vi "TTM.vi"() -> ()   [LabVIEW 2009]
doc: "This is the Target Temperature Monitoring module (TTM).\nIts job is to read all temperature measurement devices and report back the information."
uses:
  TTM Global.vi
panel:
  in  "Read LakeShore":bool
  in  "Read ITC4":bool
  in  "Read He4 Manometer":bool
  in  "Read He3 Manometer":bool
  in  "He4 Range":enum32{"X 1", "X 0.1", "X 0.01", "X 0.001"}(ring)=enum."X 0.01"
  in  "He3 Range":i32(ring)=2 items=["range X0.01", "range X0.1", "range X1"]
  out "TTM Message Type":T1(ring)=enum."He3Range="
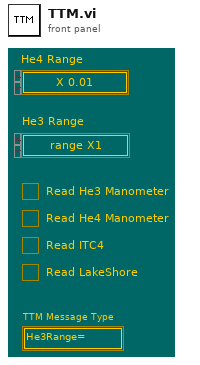
[diagram p1: front panel]
types:
  T1 = enum16{"No Message", "Bad Message", "He3Range=", "He4Range=", "GenEvent=", "Ping=", "Stop"}
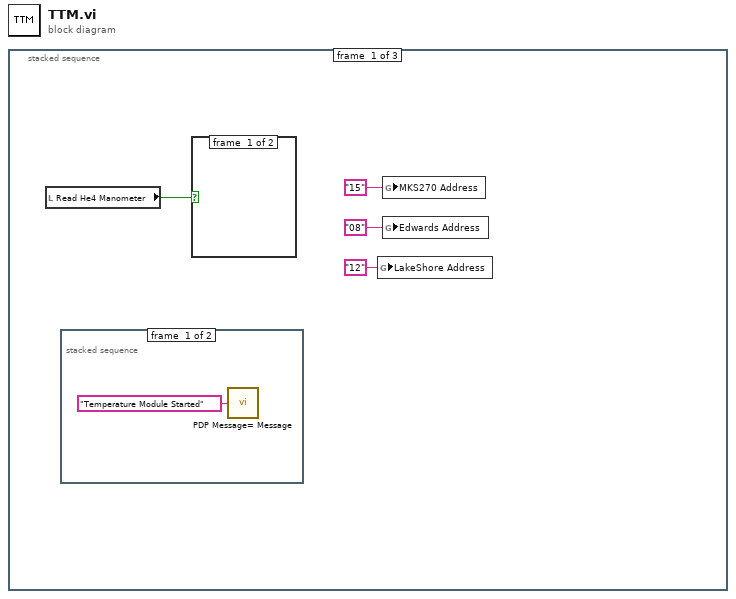
[diagram p0: block diagram]
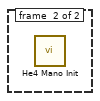
[diagram p2: hidden frame]
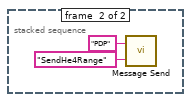
[diagram p3: hidden frame]
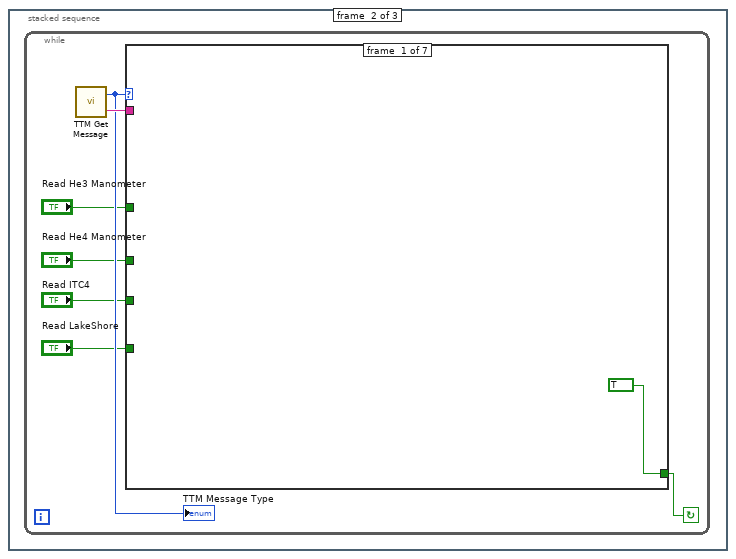
[diagram p4: hidden frame]
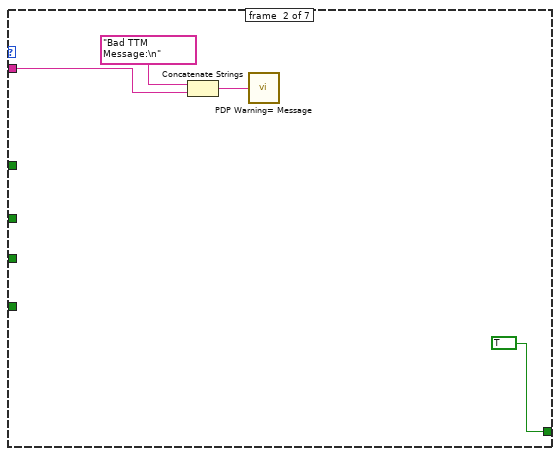
[diagram p5: hidden frame]
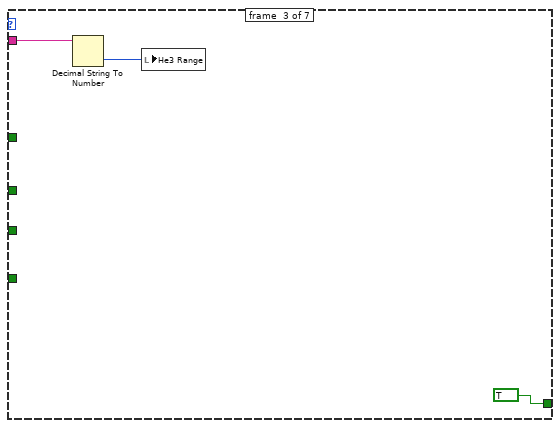
[diagram p6: hidden frame]
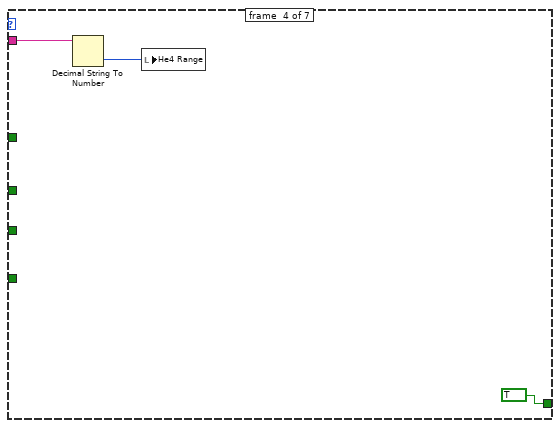
[diagram p7: hidden frame]
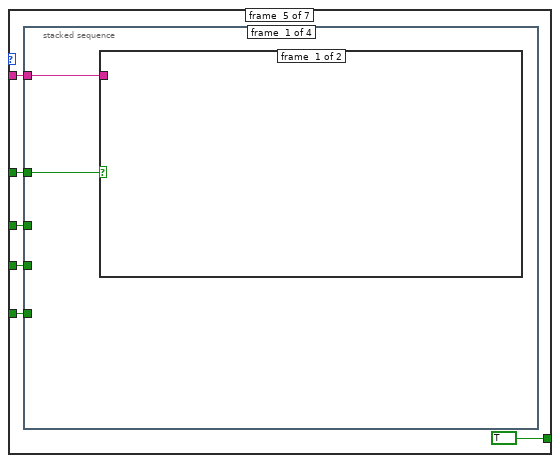
[diagram p8: hidden frame]
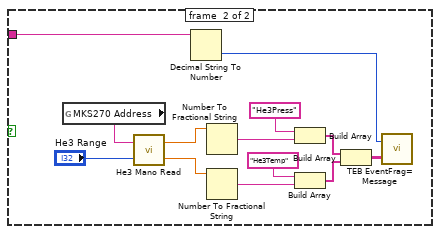
[diagram p9: hidden frame]
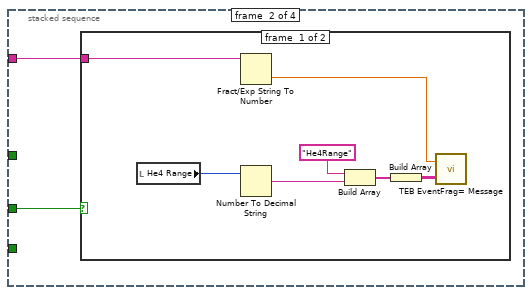
[diagram p10: hidden frame]
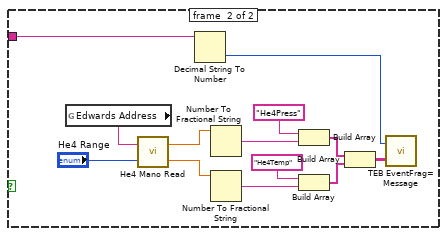
[diagram p11: hidden frame]
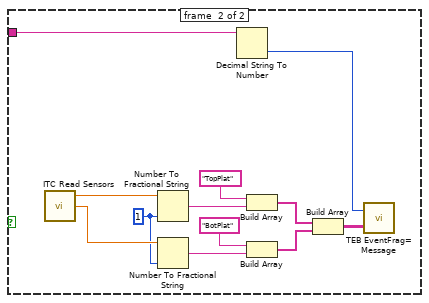
[diagram p13: hidden frame]
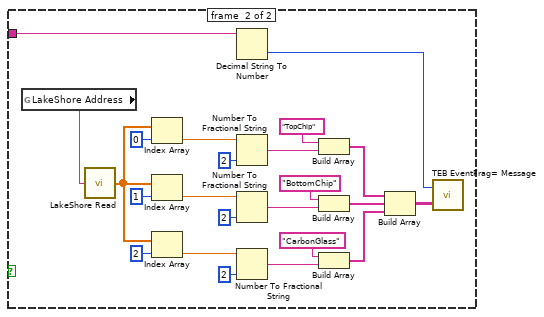
[diagram p15: hidden frame]
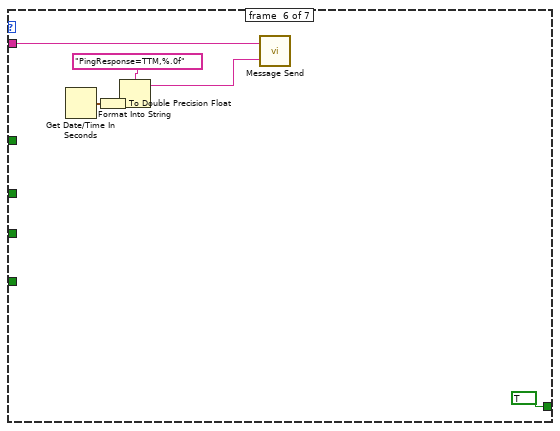
[diagram p16: hidden frame]
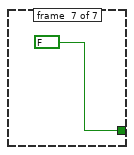
[diagram p17: hidden frame]
diagram:
  n1 = stacked-sequence {
    frame #0 {
      n2 = local read "Read He4 Manometer"() -> (w1:bool)
      n3 = stacked-sequence {
        frame #0 {
          n4 = call "PDP Message= Message.vi"("Message"="Temperature Module Started") -> ()
        }
        frame #1 {
          n5 = call "Message Send.vi"("Message"="SendHe4Range", "Destination"="PDP") -> ()
        }
      }
      n6 = case shown="True" w1 {
        frame #0 {
        }
        frame #1 {
          n7 = call "He4 Mano Init.vi"() -> ()  [unwired: 1 in]
        }
      }
      n8 = global write "TTM Global.vi" "LakeShore Address"("12" ("Edwards Address")) -> ()
      n9 = global write "TTM Global.vi" "MKS270 Address"("15" ("MKS270 Address")) -> ()
      n10 = global write "TTM Global.vi" "Edwards Address"("08" ("Edwards Address")) -> ()
    }
    frame #1 {
      n11 = while {
        stop <- w13 continue-if-true
        n12 = call "TTM Get Message.vi"() -> ("Text"=w14:string, "TTM Message Type"=w12:T1)
        "TTM Message Type" <- w12
        n13 = case shown="\"GenEvent=\"" w12 {
          tunnel: w14 -> [_ w19 w21 w24 w31 w109 _]
          tunnel: [TRUE TRUE TRUE TRUE TRUE TRUE FALSE] -> w13
          tunnel: "Read He3 Manometer" -> [_ _ _ _ w29 _ _]
          tunnel: "Read He4 Manometer" -> [_ _ _ _ w28 _ _]
          tunnel: "Read ITC4" -> [_ _ _ _ w27 _ _]
          tunnel: "Read LakeShore" -> [_ _ _ _ w26 _ _]
          frame #0 {
          }
          frame #1 {
            n14 = Concatenate Strings("Bad TTM Message:\n", w19) -> (w17:string)
            n15 = call "PDP Warning= Message.vi"("Message"=w17) -> ()
          }
          frame #2 {
            n16 = Decimal String To Number(string=w21) -> (number=w20:i32)  [unwired: 2 in, 1 out]
            n17 = local write "He3 Range"(w20) -> ()
          }
          frame #3 {
            n18 = Decimal String To Number(string=w24) -> (number=w23:i32)  [unwired: 2 in, 1 out]
            n19 = local write "He4 Range"(w23) -> ()
          }
          frame #4 {
            n20 = stacked-sequence {
              tunnel: w31 -> [w33 w48 w70 w84]
              tunnel: w29 -> [w32 _ _ _]
              tunnel: w28 -> [_ w47 _ _]
              tunnel: w27 -> [_ _ w69 _]
              tunnel: w26 -> [_ _ _ w83]
              frame #0 {
                n21 = case shown="True" w32 {
                  tunnel: w33 -> [_ w46]
                  frame #0 {
                  }
                  frame #1 {
                    n22 = global read "TTM Global.vi" "MKS270 Address"() -> (w35:string)
                    n23 = call "He3 Mano Read.vi"("Range"="He3 Range", "GPIB Address"=w35) -> ("3He Temp (K)"=w37:dbl, "3He Pressure (Torr)"=w36:dbl)
                    n24 = Decimal String To Number(string=w46) -> (number=w45:i32)  [unwired: 2 in, 1 out]
                    n25 = Number To Fractional String(number=w36) -> (F-format string=w38:string)  [unwired: 3 in]
                    n26 = Number To Fractional String(number=w37) -> (F-format string=w42:string)  [unwired: 3 in]
                    n27 = Build Array("He3Press", w38) -> (w39:string[])
                    n28 = Build Array("He3Temp", w42) -> (w43:string[])
                    n29 = Build Array(w39, w43) -> (w44:string[][])
                    n30 = call "TEB EventFrag= Message.vi"("Event Fragment(s)"=w44, "Event Number"=w45) -> ()
                  }
                }
              }
              frame #1 {
                n31 = case shown="True" w47 {
                  tunnel: w48 -> [w52 w68]
                  frame #0 {
                    n32 = local read "He4 Range"() -> (w50:enum32{"X 1", "X 0.1", "X 0.01", "X 0.001"})
                    n33 = Fract/Exp String To Number(string=w52) -> (number=w53:dbl)  [unwired: 3 in, 1 out]
                    n34 = Number To Decimal String(number=w50) -> (decimal integer string=w49:string)  [unwired: 1 in]
                    n35 = Build Array("He4Range", w49) -> (w55:string[])
                    n36 = Build Array(w55) -> (w51:string[][])
                    n37 = call "TEB EventFrag= Message.vi"("Event Fragment(s)"=w51, "Event Number"=w53) -> ()
                  }
                  frame #1 {
                    n38 = global read "TTM Global.vi" "Edwards Address"() -> (w57:string)
                    n39 = call "He4 Mano Read.vi"("Range"="He4 Range", "GPIB Address"=w57) -> ("Temperature (K)"=w59:dbl, "Vapor pressure (torr)"=w58:dbl)
                    n40 = Decimal String To Number(string=w68) -> (number=w67:i32)  [unwired: 2 in, 1 out]
                    n41 = Number To Fractional String(number=w58) -> (F-format string=w60:string)  [unwired: 3 in]
                    n42 = Number To Fractional String(number=w59) -> (F-format string=w64:string)  [unwired: 3 in]
                    n43 = Build Array("He4Press", w60) -> (w61:string[])
                    n44 = Build Array("He4Temp", w64) -> (w65:string[])
                    n45 = Build Array(w61, w65) -> (w66:string[][])
                    n46 = call "TEB EventFrag= Message.vi"("Event Fragment(s)"=w66, "Event Number"=w67) -> ()
                  }
                }
              }
              frame #2 {
                n47 = case shown="True" w69 {
                  tunnel: w70 -> [_ w82]
                  frame #0 {
                  }
                  frame #1 {
                    w71 = i16 1 ("precision (6)")
                    n48 = call "ITC Read Sensors.vi"() -> ("Sensor 2"=w73:dbl, "Sensor 1"=w72:dbl)  [unwired: 1 in]
                    n49 = Number To Fractional String(number=w72, precision (6)=w71) -> (F-format string=w75:string)  [unwired: 2 in]
                    n50 = Number To Fractional String(number=w73, precision (6)=w71) -> (F-format string=w74:string)  [unwired: 2 in]
                    n51 = Decimal String To Number(string=w82) -> (number=w81:i32)  [unwired: 2 in, 1 out]
                    n52 = Build Array("TopPlat", w75) -> (w77:string[])
                    n53 = Build Array("BotPlat", w74) -> (w76:string[])
                    n54 = Build Array(w77, w76) -> (w80:string[][])
                    n55 = call "TEB EventFrag= Message.vi"("Event Fragment(s)"=w80, "Event Number"=w81) -> ()
                  }
                }
              }
              frame #3 {
                n56 = case shown="True" w83 {
                  tunnel: w84 -> [_ w107]
                  frame #0 {
                  }
                  frame #1 {
                    n57 = global read "TTM Global.vi" "LakeShore Address"() -> (w89:string)
                    n58 = call "LakeShore Read.vi"("Address"=w89) -> ("subarray"=w88:dbl[])
                    n59 = Index Array(array=w88, index=0) -> (element=w102:dbl)
                    n60 = Index Array(array=w88, index=1) -> (element=w98:dbl)
                    n61 = Index Array(array=w88, index=2) -> (element=w97:dbl)
                    n62 = Decimal String To Number(string=w107) -> (number=w106:i32)  [unwired: 2 in, 1 out]
                    n63 = Number To Fractional String(number=w102, precision (6)=i16 2) -> (F-format string=w100:string)  [unwired: 2 in]
                    n64 = Number To Fractional String(number=w98, precision (6)=i16 2) -> (F-format string=w93:string)  [unwired: 2 in]
                    n65 = Number To Fractional String(number=w97, precision (6)=i16 2) -> (F-format string=w92:string)  [unwired: 2 in]
                    n66 = Build Array("TopChip", w100) -> (w103:string[])
                    n67 = Build Array("BottomChip", w93) -> (w90:string[])
                    n68 = Build Array("CarbonGlass", w92) -> (w91:string[])
                    n69 = Build Array(w103, w90, w91) -> (w105:string[][])
                    n70 = call "TEB EventFrag= Message.vi"("Event Fragment(s)"=w105, "Event Number"=w106) -> ()
                  }
                }
              }
            }
          }
          frame #5 {
            n71 = Get Date/Time In Seconds() -> (seconds since 1Jan1904=w108:timestamp)
            n72 = To Double Precision Float(number=w108) -> (double precision float=w111:dbl)
            n73 = Format Into String(format string="PingResponse=TTM,%.0f", w111) -> (resulting string=w110:string)  [unwired: 2 in, 1 out]
            n74 = call "Message Send.vi"("Message"=w110, "Destination"=w109) -> ()
          }
          frame #6 {
          }
        }
      }
    }
    frame #2 {
    }
  }
